vi "GetAttributePaths.vi"() -> ()   [LabVIEW 2012]
doc: "SciScan 1.2 160622"
uses:
  <vilib>/xml/NI_XML.lvlib
  <resource>/objmgr/DOMUserDefRef.rc
panel:
  out "error out":errorcluster
  out "XML":string
  out "Array 4":string[](array[string])
  out "Array 3":string[](array[string])
  in  "XML File Path":path
  out "Array 2":string[][](array[string])
  in  "DOM document out":refnum<k20>
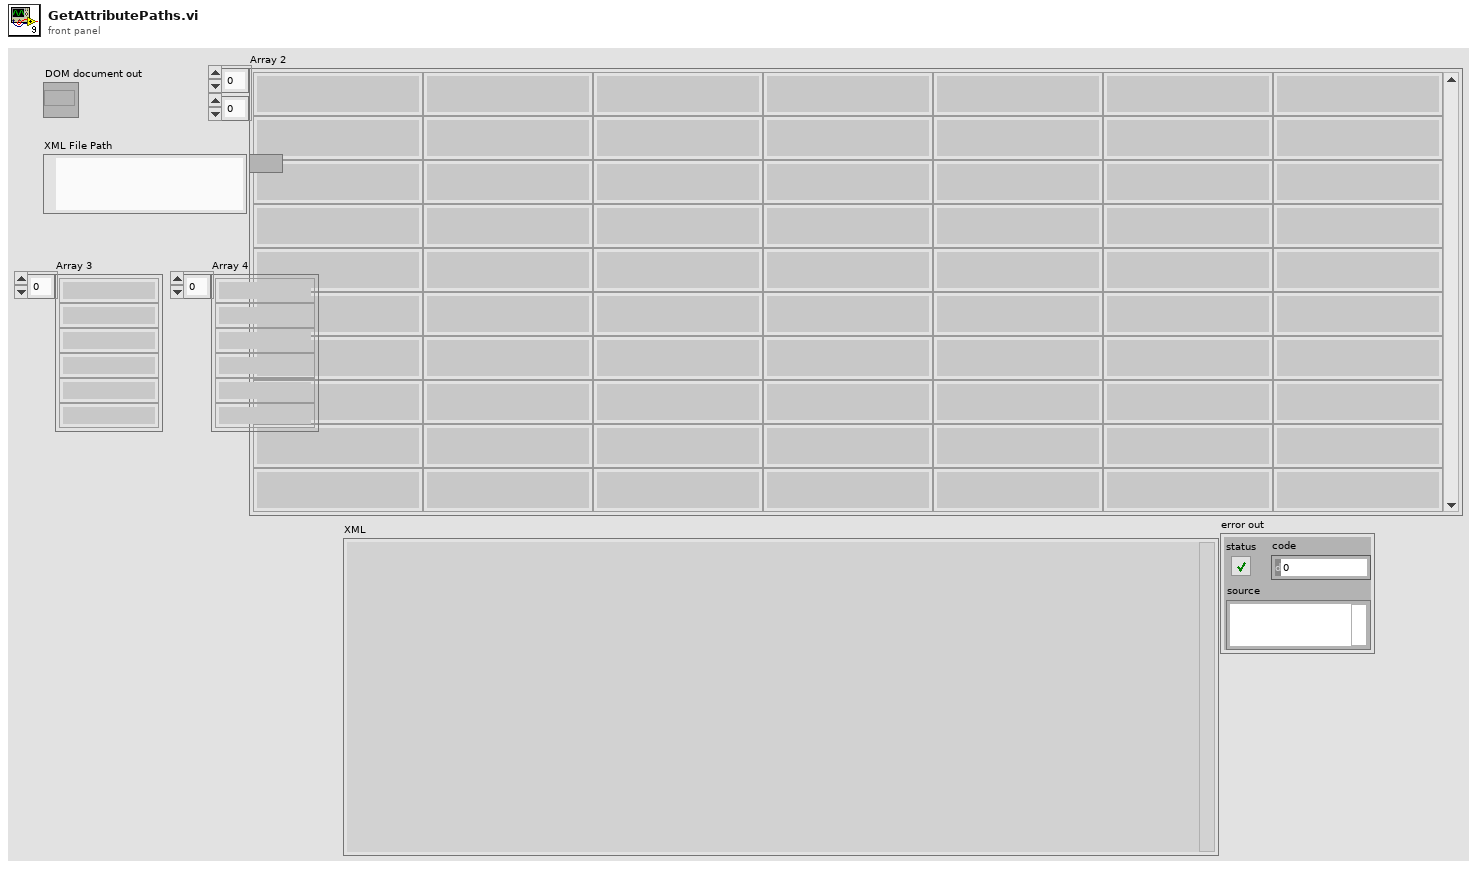
[diagram p1: front panel]
types:
  T1 = cluster{"Node":refnum<k20>, "Node Reg":refnum<k20>}
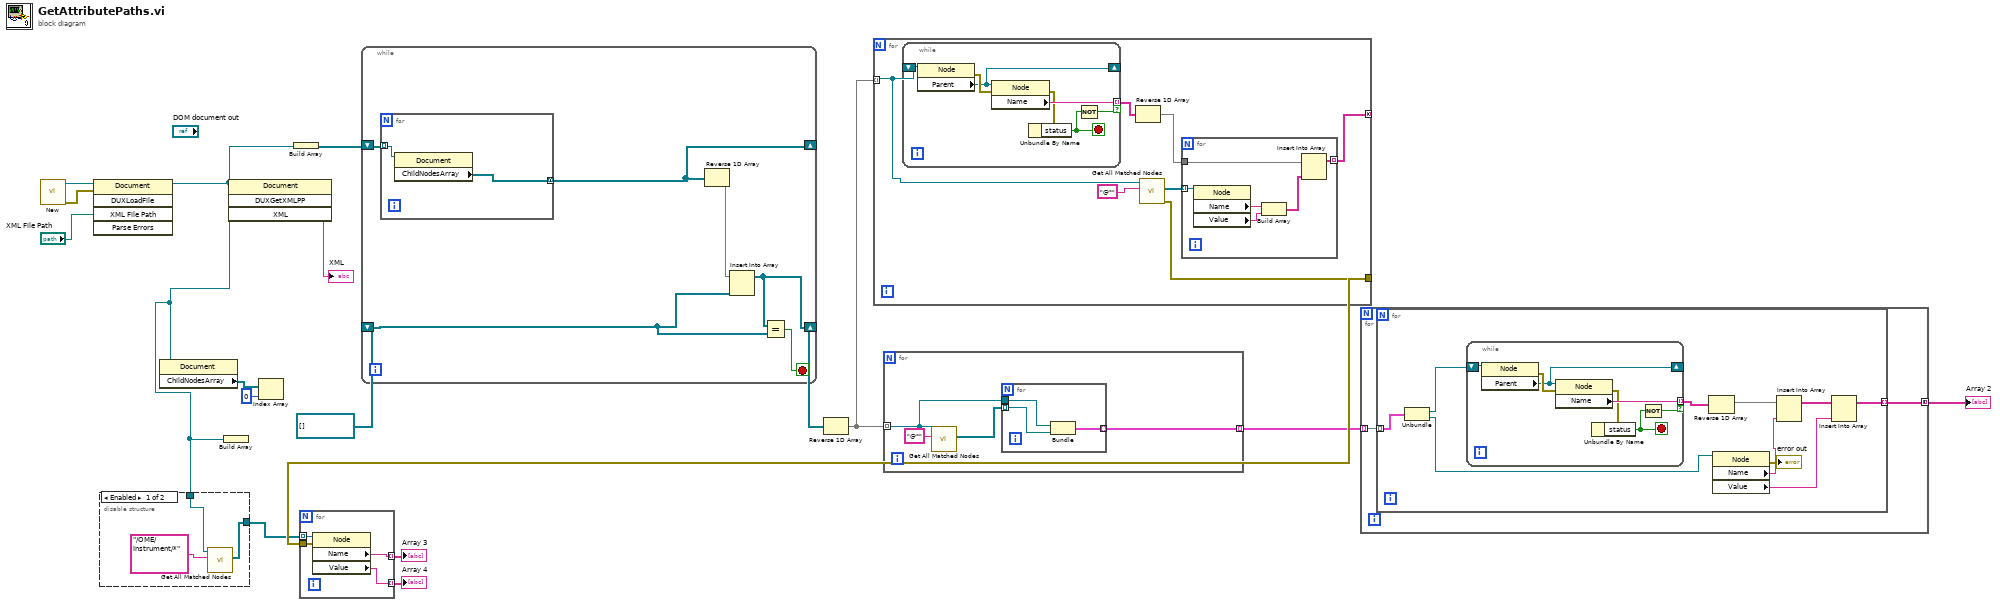
[diagram p0: block diagram]
diagram:
  n1 = call <vilib>:"New.vi"() -> ("error out"=w13:errorcluster, "DOM document out"=w11:refnum<k20>)  [unwired: 8 in]
  n2 = invoke class="Document" method="DUXLoadFile"(reference=w11, error in=w13, "XML File Path"="XML File Path") -> (reference out=w4:refnum<k20>)  [unwired: 2 in, 4 out]
  n3 = disable-structure shown="Enabled" {
    disable-tunnel: [w19 w21] -> w5
    disable-tunnel: w4 -> [w20 w21]
    frame Enabled {
      n4 = call <vilib>:"Get All Matched Nodes.vi"("XPath expression"="/OME/Instrument/*", "node in"=w20) -> ("node result array"=w19:refnum<k20>[])  [unwired: 7 in, 2 out]
    }
    frame Disabled {
    }
  }
  n5 = property class="Document"(reference=w4) -> ("ChildNodesArray"=w9:refnum<k20>[])  [unwired: 1 in, 2 out]
  n6 = Build Array(w4) -> ()  [unwired: 1 out]
  n7 = invoke class="Document" method="DUXGetXMLPP"(reference=w4) -> ("XML"=→"XML":string)  [unwired: 3 in, 3 out]
  n8 = Index Array(array=w9, index=0) -> ()  [unwired: 1 out]
  n9 = Build Array(w4) -> (w16:refnum<k20>[])
  n10 = while {
    shift-right: [w23] -> w17
    shift-left: refnum<k20>[] [] -> [w22]
    shift-right: [w25] -> _
    shift-left: w16 -> [w24]
    stop <- w27 stop-if-true
    n11 = for {
      tunnel: [w28] -> w25 mode=concatenating
      tunnel: w24 -> [w29] mode=indexing
      n12 = property class="Document"(reference=w29) -> ("ChildNodesArray"=w28:refnum<k20>[])  [unwired: 1 in, 2 out]
    }
    n13 = Reverse 1D Array(array=w25) -> (reversed array=w26:refnum<k20>[])
    n14 = Insert Into Array(array=w26, new element=w22) -> (w23:refnum<k20>[])  [unwired: 1 in]
    n15 = Equal?(x=w23, y=w22) -> (x = y?=w27:bool)
  }
  n16 = Reverse 1D Array(array=w17) -> (reversed array=w14:refnum<k20>[])
  n17 = for {
    tunnel: w14 -> [w31] mode=indexing
    tunnel: [w32] -> _ mode=concatenating
    tunnel: [w30] -> w10
    n18 = while {
      tunnel: [w48] -> w36 mode=indexing if=w45
      shift-right: [w43] -> _
      shift-left: w31 -> [w49]
      stop <- w44 stop-if-true
      n19 = property class="Node"(reference=w49) -> (error out=w47:errorcluster, "Parent"=w43:refnum<k20>)  [unwired: 1 in, 1 out]
      n20 = property class="Node"(reference=w43, error in=w47) -> (error out=w46:errorcluster, "Name"=w48:string)  [unwired: 1 out]
      n21 = Unbundle By Name(w46) -> ("status"=w44:bool)
      n22 = Not(x=w44) -> (.not. x?=w45:bool)
    }
    n23 = Reverse 1D Array(array=w36) -> (reversed array=w33:string[])
    n24 = call <vilib>:"Get All Matched Nodes.vi"("XPath expression"="@*", "node in"=w31) -> ("error out"=w30:errorcluster, "node result array"=w34:refnum<k20>[])  [unwired: 7 in, 1 out]
    n25 = for {
      tunnel: w34 -> [w42] mode=indexing
      tunnel: w33 -> [w39]
      tunnel: [w37] -> w32 mode=indexing
      n26 = property class="Node"(reference=w42) -> ("Name"=w41:string, "Value"=w40:string)  [unwired: 1 in, 2 out]
      n27 = Build Array(w41, w40) -> (w38:string[])
      n28 = Insert Into Array(array=w39, new element=w38) -> (w37:string[])  [unwired: 1 in]
    }
  }
  n29 = for {
    tunnel: w5 -> [w53] mode=indexing
    tunnel: [w52] -> w6 mode=indexing
    tunnel: [w51] -> w7 mode=indexing
    tunnel: w10 -> [w50]
    n30 = property class="Node"(reference=w53, error in=w50) -> ("Name"=w51:string, "Value"=w52:string)  [unwired: 2 out]
  }
  "Array 3" <- w7
  "Array 4" <- w6
  n31 = for {
    tunnel: w14 -> [w55] mode=indexing
    tunnel: [w54] -> w2 mode=indexing
    n32 = call <vilib>:"Get All Matched Nodes.vi"("XPath expression"="@*", "node in"=w55) -> ("node result array"=w56:refnum<k20>[])  [unwired: 7 in, 2 out]
    n33 = for {
      tunnel: w56 -> [w60] mode=indexing
      tunnel: w55 -> [w59]
      tunnel: [w58] -> w54 mode=indexing
      n34 = Bundle("Node"=w59, "Node Reg"=w60) -> (w58:T1)  [unwired: 1 in]
    }
  }
  n35 = for {
    tunnel: w2 -> [w62] mode=indexing
    tunnel: [w61] -> w1 mode=concatenating
    n36 = for {
      tunnel: w62 -> [w72] mode=indexing
      tunnel: [w64] -> w61 mode=indexing
      n37 = Unbundle(w72) -> ("Node"=w71:refnum<k20>, "Node Reg"=w68:refnum<k20>)
      n38 = while {
        tunnel: [w78] -> w70 mode=indexing if=w75
        shift-right: [w73] -> _
        shift-left: w71 -> [w79]
        stop <- w74 stop-if-true
        n39 = property class="Node"(reference=w79) -> (error out=w77:errorcluster, "Parent"=w73:refnum<k20>)  [unwired: 1 in, 1 out]
        n40 = property class="Node"(reference=w73, error in=w77) -> (error out=w76:errorcluster, "Name"=w78:string)  [unwired: 1 out]
        n41 = Unbundle By Name(w76) -> ("status"=w74:bool)
        n42 = Not(x=w74) -> (.not. x?=w75:bool)
      }
      n43 = Reverse 1D Array(array=w70) -> (reversed array=w69:string[])
      n44 = property class="Node"(reference=w68) -> (error out=→"error out":errorcluster, "Name"=w67:string, "Value"=w65:string)  [unwired: 1 in, 1 out]
      n45 = Insert Into Array(array=w69, new element=w67) -> (w66:string[])  [unwired: 1 in]
      n46 = Insert Into Array(array=w66, new element=w65) -> (w64:string[])  [unwired: 1 in]
    }
  }
  "Array 2" <- w1
